vi "IMAQDevice.ReadIniFile.vi"(1 "ObjectName":string, 3 "Path":path, 5 "error in (no error)":errorcluster) -> (7 "Rotation":dbl, 8 "TimeOut":i32, 9 "Mirror":string, 10 "OffsetFromLeft":i32, 11 "HorizontalPixelPerMm":dbl, 12 "OffsetFromTop":i32, 13 "VerticalPixelPerMm":dbl, 14 "Serial Number":string, 15 "start sequence array":cluster{"Command":string, "Value":string}[](array[cluster]), 16 "Camera-Names":string[](array[string]), 17 "Grid":T1, 18 "GridR":T2, 19 "error out":errorcluster)   [LabVIEW 2014, in "IMAQDevice.lvlib"]
uses:
  IMAQDevice.lvlib
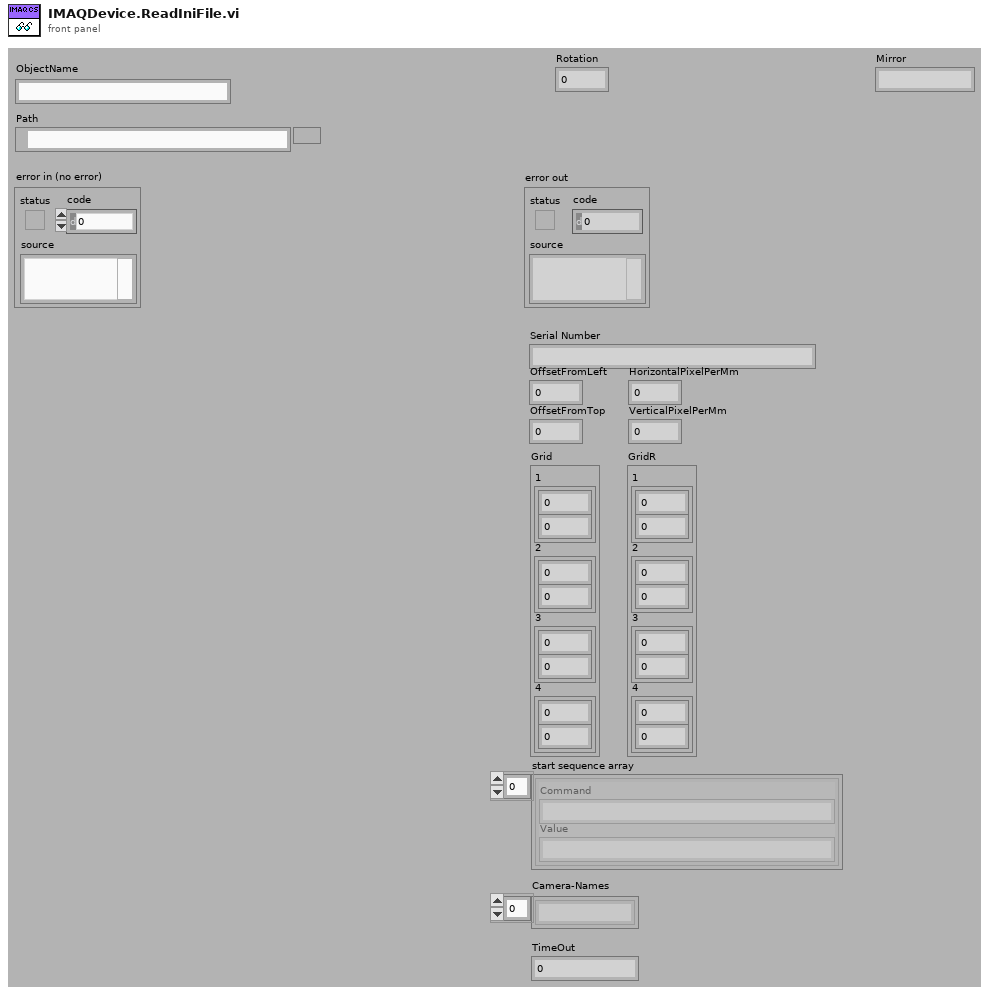
[diagram p1: front panel]
types:
  T1 = cluster{"1":cluster{i32, i32}, "2":cluster{i32, i32}, "3":cluster{i32, i32}, "4":cluster{i32, i32}}
  T2 = cluster{"1":cluster{dbl, dbl}, "2":cluster{dbl, dbl}, "3":cluster{dbl, dbl}, "4":cluster{dbl, dbl}}
  T3 = cluster{cluster{i32, i32}, cluster{i32, i32}, cluster{i32, i32}, cluster{i32, i32}}
  T4 = cluster{cluster{dbl, dbl}, cluster{dbl, dbl}, cluster{dbl, dbl}, cluster{dbl, dbl}}
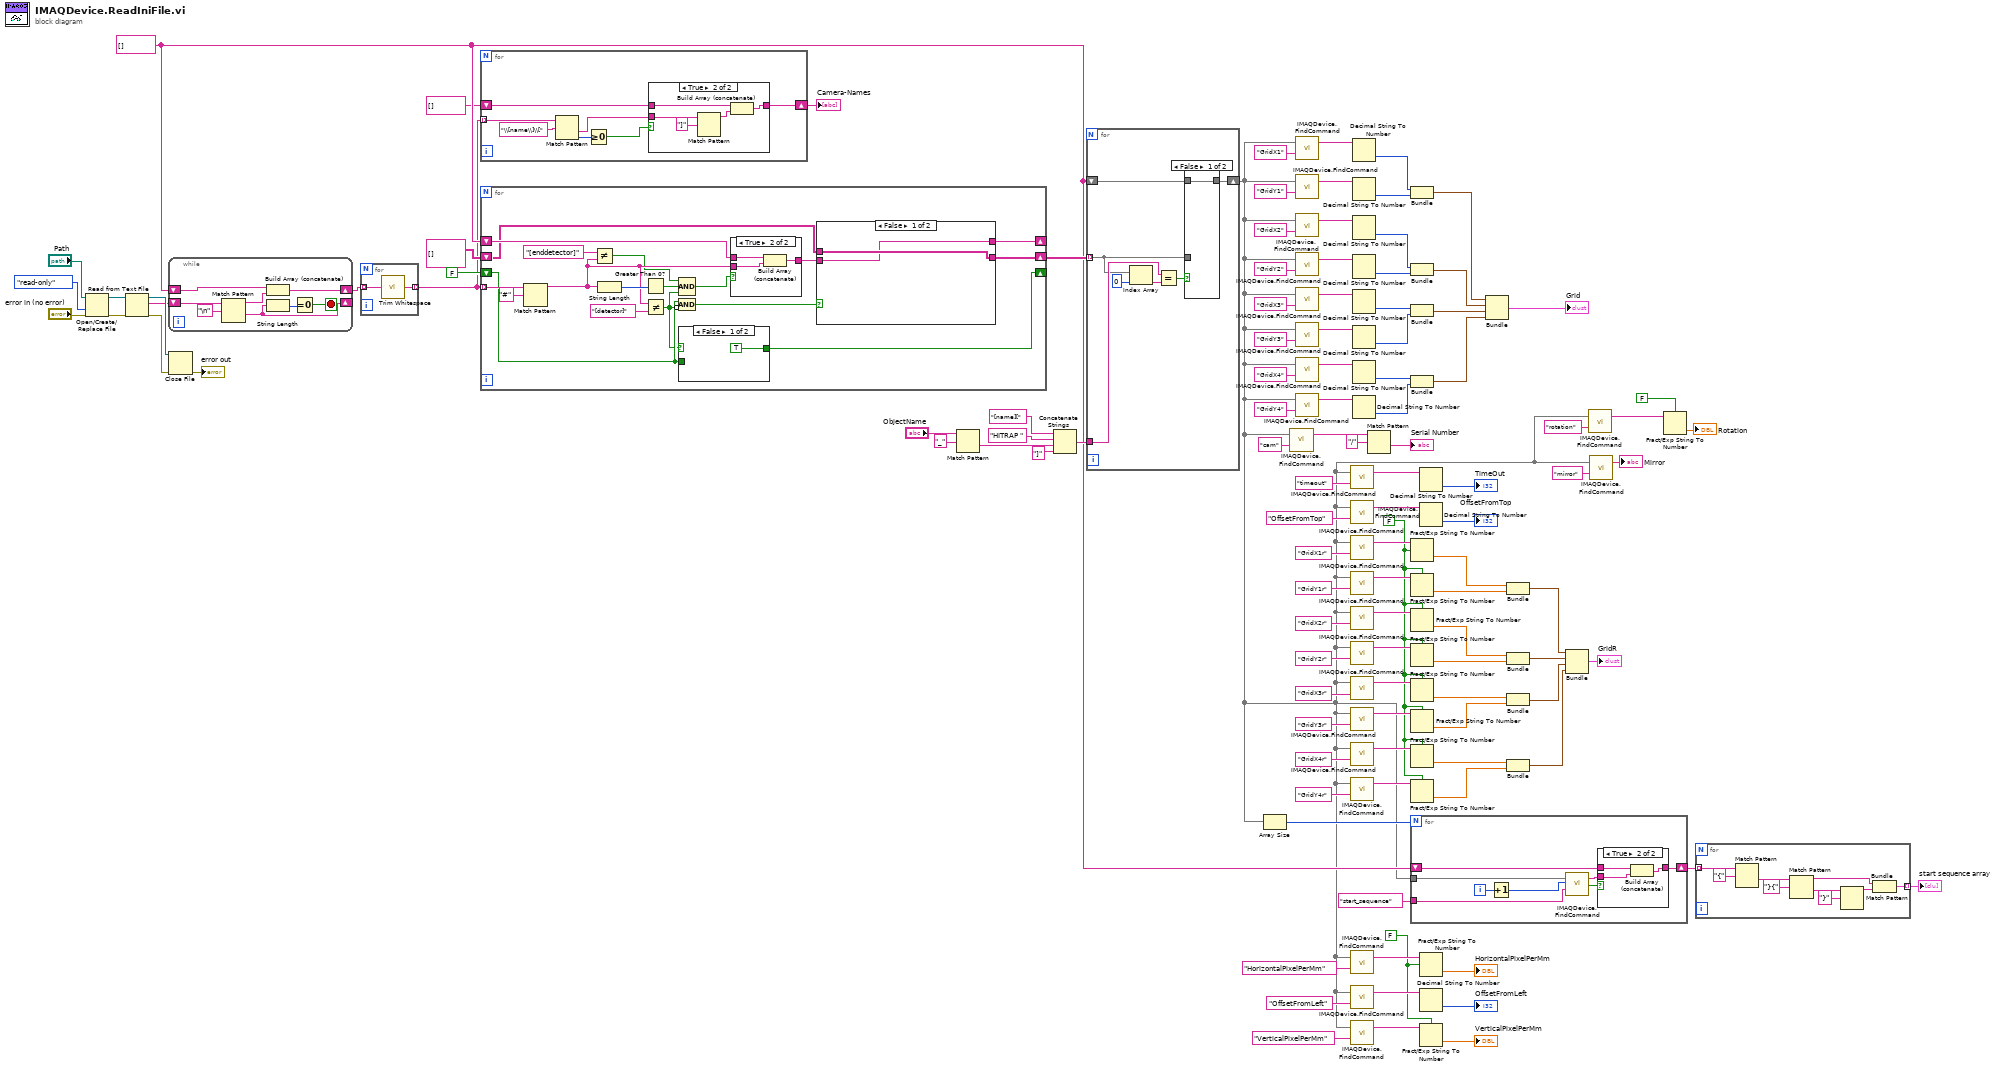
[diagram p0: block diagram]
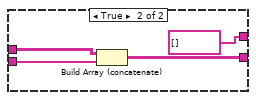
[diagram p6: hidden frame]
diagram:
  w8 = FALSE ("use system decimal point (T)")
  w9 = FALSE ("use system decimal point (T)")
  w27 = string[] []
  n1 = Open/Create/Replace File(file path (use dialog)="Path", error in="error in (no error)", access (0:read/write)=enum16{"read/write", "read-only", "write-only"}."read-only") -> (refnum out=w111:refnum<file>, error out=w110:errorcluster)  [unwired: 3 in, 1 out]
  n2 = Read from Text File(file (use dialog)=w111, error in=w110) -> (refnum out=w109:refnum<file>, text=w107:string, error out=w108:errorcluster)  [unwired: 2 in, 1 out]
  n3 = while {
    shift-right: [w117] -> _
    shift-left: w107 -> [w122]
    shift-right: [w119] -> w19
    shift-left: w27 -> [w120]
    stop <- w115 stop-if-true
    n4 = Match Pattern(string=w122, regular expression="\n") -> (before substring=w118:string, after substring=w117:string)  [unwired: 1 in, 2 out]
    n5 = Build Array (concatenate)(w120, w118) -> (w119:string[])
    n6 = String Length(string=w117) -> (length=w116:i32)
    n7 = Equal To 0?(x=w116) -> (x = 0?=w115:bool)
  }
  n8 = Close File(refnum=w109, error in=w108) -> (error out=→"error out":errorcluster)  [unwired: 1 out]
  n9 = for {
    tunnel: w19 -> [w124] mode=indexing
    tunnel: [w123] -> w18 mode=indexing
    n10 = call <vilib>:"Trim Whitespace.vi"("string"=w124) -> ("trimmed string"=w123:string)  [unwired: 1 in]
  }
  n11 = for {
    tunnel: w18 -> [w131] mode=indexing
    shift-right: [w128] -> w20
    shift-left: string[] [] -> [w129]
    n12 = Match Pattern(string=w131, regular expression="\\[name\\]\\[") -> (after substring=w126:string, offset past match=w127:i32)  [unwired: 1 in, 2 out]
    n13 = Greater Or Equal To 0?(x=w127) -> (x >= 0?=w125:bool)
    n14 = case shown="True" w125 {
      tunnel: w129 -> [w132 w137]
      tunnel: [w132 w136] -> w128
      tunnel: w126 -> [_ w134]
      frame False {
      }
      frame True {
        n15 = Match Pattern(string=w134, regular expression="]") -> (before substring=w133:string)  [unwired: 1 in, 3 out]
        n16 = Build Array (concatenate)(w137, w133) -> (w136:string[])
      }
    }
  }
  "Camera-Names" <- w20
  n17 = for {
    tunnel: w18 -> [w145] mode=indexing
    shift-right: [w147] -> w103
    shift-left: string[][] [] -> [w148]
    shift-right: [w144] -> _
    shift-left: w27 -> [w150]
    shift-right: [w143] -> _
    shift-left: FALSE -> [w142]
    n18 = Match Pattern(string=w145, regular expression="#") -> (before substring=w139:string)  [unwired: 1 in, 3 out]
    n19 = Not Equal?(x="[enddetector]" ("y"), y=w139) -> (x != y?=w138:bool)
    n20 = String Length(string=w139) -> (length=w155:i32)
    n21 = Greater Than 0?(x=w155) -> (x > 0?=w151:bool)
    n22 = Not Equal?(x=w139, y="[detector]") -> (x != y?=w141:bool)
    n23 = Compound Arithmetic op=AND(w138, w151, w141) -> (w152:bool)
    n24 = Compound Arithmetic op=AND(w142, invert w141) -> (w149:bool)
    n25 = case shown="False" w141 {
      tunnel: [TRUE w157] -> w143
      tunnel: w142 -> [_ w157]
      frame False {
      }
      frame True {
      }
    }
    n26 = case shown="True" w152 {
      tunnel: w139 -> [_ w167]
      tunnel: w150 -> [w164 w166]
      tunnel: [w164 w165] -> w146
      frame False {
      }
      frame True {
        n27 = Build Array (concatenate)(w166, w167) -> (w165:string[])
      }
    }
    n28 = case shown="False" w149 {
      tunnel: w148 -> [w159 w163]
      tunnel: [w159 w162] -> w147
      tunnel: w146 -> [w158 w161]
      tunnel: [w158 string[] []] -> w144
      frame False {
      }
      frame True {
        n29 = Build Array (concatenate)(w163, w161) -> (w162:string[][])
      }
    }
  }
  n30 = Match Pattern(string="ObjectName", regular expression="_") -> (after substring=w15:string)  [unwired: 1 in, 3 out]
  n31 = Concatenate Strings("[name][" ("string"), "HITRAP ", w15, "]" ("string")) -> (w102:string)
  n32 = for {
    tunnel: w103 -> [w169] mode=indexing
    tunnel: w102 -> [w172]
    shift-right: [w168] -> w4
    shift-left: w27 -> [w170]
    n33 = Index Array(array=w169, index=0) -> (element=w173:string)
    n34 = Equal?(x=w172, y=w173) -> (x = y?=w171:bool)
    n35 = case shown="False" w171 {
      tunnel: w170 -> [w175 _]
      tunnel: w169 -> [_ w176]
      tunnel: [w175 w176] -> w168
      frame False {
      }
      frame True {
      }
    }
  }
  n36 = Array Size(array=w4) -> (size(s)=w29:i32)
  n37 = call "IMAQDevice.FindCommand.vi"("Command Array"=w4, "Search String"="cam") -> ("Found Result"=w23:string)  [unwired: 16 in, 1 out]
  n38 = call "IMAQDevice.FindCommand.vi"("Command Array"=w4, "Search String"="GridX1") -> ("Found Result"=w79:string)  [unwired: 16 in, 1 out]
  n39 = call "IMAQDevice.FindCommand.vi"("Command Array"=w4, "Search String"="GridY1") -> ("Found Result"=w78:string)  [unwired: 16 in, 1 out]
  n40 = call "IMAQDevice.FindCommand.vi"("Command Array"=w4, "Search String"="GridX2") -> ("Found Result"=w77:string)  [unwired: 16 in, 1 out]
  n41 = call "IMAQDevice.FindCommand.vi"("Command Array"=w4, "Search String"="GridY2") -> ("Found Result"=w76:string)  [unwired: 16 in, 1 out]
  n42 = call "IMAQDevice.FindCommand.vi"("Command Array"=w4, "Search String"="GridX3") -> ("Found Result"=w75:string)  [unwired: 16 in, 1 out]
  n43 = call "IMAQDevice.FindCommand.vi"("Command Array"=w4, "Search String"="GridY3") -> ("Found Result"=w74:string)  [unwired: 16 in, 1 out]
  n44 = call "IMAQDevice.FindCommand.vi"("Command Array"=w4, "Search String"="GridX4") -> ("Found Result"=w73:string)  [unwired: 16 in, 1 out]
  n45 = call "IMAQDevice.FindCommand.vi"("Command Array"=w4, "Search String"="GridY4") -> ("Found Result"=w72:string)  [unwired: 16 in, 1 out]
  n46 = call "IMAQDevice.FindCommand.vi"("Command Array"=w4, "Search String"="timeout") -> ("Found Result"=w11:string)  [unwired: 16 in, 1 out]
  n47 = call "IMAQDevice.FindCommand.vi"("Command Array"=w4, "Search String"="OffsetFromTop") -> ("Found Result"=w96:string)  [unwired: 16 in, 1 out]
  n48 = call "IMAQDevice.FindCommand.vi"("Command Array"=w4, "Search String"="GridX1r") -> ("Found Result"=w50:string)  [unwired: 16 in, 1 out]
  n49 = call "IMAQDevice.FindCommand.vi"("Command Array"=w4, "Search String"="GridY1r") -> ("Found Result"=w49:string)  [unwired: 16 in, 1 out]
  n50 = call "IMAQDevice.FindCommand.vi"("Command Array"=w4, "Search String"="GridX2r") -> ("Found Result"=w48:string)  [unwired: 16 in, 1 out]
  n51 = call "IMAQDevice.FindCommand.vi"("Command Array"=w4, "Search String"="GridY2r") -> ("Found Result"=w47:string)  [unwired: 16 in, 1 out]
  n52 = call "IMAQDevice.FindCommand.vi"("Command Array"=w4, "Search String"="GridX3r") -> ("Found Result"=w46:string)  [unwired: 16 in, 1 out]
  n53 = call "IMAQDevice.FindCommand.vi"("Command Array"=w4, "Search String"="GridY3r") -> ("Found Result"=w45:string)  [unwired: 16 in, 1 out]
  n54 = call "IMAQDevice.FindCommand.vi"("Command Array"=w4, "Search String"="GridX4r") -> ("Found Result"=w44:string)  [unwired: 16 in, 1 out]
  n55 = call "IMAQDevice.FindCommand.vi"("Command Array"=w4, "Search String"="GridY4r") -> ("Found Result"=w43:string)  [unwired: 16 in, 1 out]
  n56 = call "IMAQDevice.FindCommand.vi"("Command Array"=w4, "Search String"="HorizontalPixelPerMm") -> ("Found Result"=w91:string)  [unwired: 16 in, 1 out]
  n57 = call "IMAQDevice.FindCommand.vi"("Command Array"=w4, "Search String"="OffsetFromLeft") -> ("Found Result"=w94:string)  [unwired: 16 in, 1 out]
  n58 = call "IMAQDevice.FindCommand.vi"("Command Array"=w4, "Search String"="VerticalPixelPerMm") -> ("Found Result"=w89:string)  [unwired: 16 in, 1 out]
  n59 = Decimal String To Number(string=w79) -> (number=w66:i32)  [unwired: 2 in, 1 out]
  n60 = Decimal String To Number(string=w78) -> (number=w65:i32)  [unwired: 2 in, 1 out]
  n61 = Decimal String To Number(string=w77) -> (number=w64:i32)  [unwired: 2 in, 1 out]
  n62 = Decimal String To Number(string=w76) -> (number=w63:i32)  [unwired: 2 in, 1 out]
  n63 = Decimal String To Number(string=w75) -> (number=w62:i32)  [unwired: 2 in, 1 out]
  n64 = Decimal String To Number(string=w74) -> (number=w61:i32)  [unwired: 2 in, 1 out]
  n65 = Decimal String To Number(string=w73) -> (number=w60:i32)  [unwired: 2 in, 1 out]
  n66 = Decimal String To Number(string=w72) -> (number=w59:i32)  [unwired: 2 in, 1 out]
  n67 = Match Pattern(string=w23, regular expression="/") -> (after substring=→"Serial Number":string)  [unwired: 1 in, 3 out]
  n68 = Bundle(w66, w65) -> (w70:cluster{i32, i32})  [unwired: 1 in]
  n69 = Bundle(w64, w63) -> (w69:cluster{i32, i32})  [unwired: 1 in]
  n70 = Bundle(w62, w61) -> (w68:cluster{i32, i32})  [unwired: 1 in]
  n71 = Bundle(w60, w59) -> (w67:cluster{i32, i32})  [unwired: 1 in]
  n72 = Fract/Exp String To Number(use system decimal point (T)=w9, string=w50) -> (number=w38:dbl)  [unwired: 2 in, 1 out]
  n73 = Fract/Exp String To Number(use system decimal point (T)=w9, string=w49) -> (number=w37:dbl)  [unwired: 2 in, 1 out]
  n74 = Fract/Exp String To Number(use system decimal point (T)=w9, string=w48) -> (number=w36:dbl)  [unwired: 2 in, 1 out]
  n75 = Fract/Exp String To Number(use system decimal point (T)=w9, string=w47) -> (number=w35:dbl)  [unwired: 2 in, 1 out]
  n76 = Fract/Exp String To Number(use system decimal point (T)=w9, string=w46) -> (number=w34:dbl)  [unwired: 2 in, 1 out]
  n77 = Fract/Exp String To Number(use system decimal point (T)=w9, string=w45) -> (number=w33:dbl)  [unwired: 2 in, 1 out]
  n78 = Fract/Exp String To Number(use system decimal point (T)=w9, string=w44) -> (number=w32:dbl)  [unwired: 2 in, 1 out]
  n79 = Fract/Exp String To Number(use system decimal point (T)=w9, string=w43) -> (number=w31:dbl)  [unwired: 2 in, 1 out]
  n80 = for {
    N: w29 -> [_]
    tunnel: w4 -> [w184]
    tunnel: "start_sequence" ("Search String") -> [w181]
    shift-right: [w178] -> w26
    shift-left: w27 -> [w179]
    i -> [w183]
    n81 = Increment(x=w183) -> (x+1=w182:i32)
    n82 = call "IMAQDevice.FindCommand.vi"("Command Array"=w184, "Sequence Number"=w182, "Search String"=w181) -> ("Found Result"=w177:string, "Found?"=w180:bool)  [unwired: 15 in]
    n83 = case shown="True" w180 {
      tunnel: w179 -> [w185 w187]
      tunnel: [w185 w188] -> w178
      tunnel: w177 -> [_ w186]
      frame False {
      }
      frame True {
        n84 = Build Array (concatenate)(w187, w186) -> (w188:string[])
      }
    }
  }
  n85 = Decimal String To Number(string=w11) -> (number=→"TimeOut":i32)  [unwired: 2 in, 1 out]
  n86 = Decimal String To Number(string=w96) -> (number=→"OffsetFromTop":i32)  [unwired: 2 in, 1 out]
  n87 = Fract/Exp String To Number(use system decimal point (T)=w8, string=w91) -> (number=→"HorizontalPixelPerMm":dbl)  [unwired: 2 in, 1 out]
  n88 = Decimal String To Number(string=w94) -> (number=→"OffsetFromLeft":i32)  [unwired: 2 in, 1 out]
  n89 = Fract/Exp String To Number(use system decimal point (T)=w8, string=w89) -> (number=→"VerticalPixelPerMm":dbl)  [unwired: 2 in, 1 out]
  n90 = Bundle(w70, w69, w68, w67) -> (→"Grid":T3)  [unwired: 1 in]
  n91 = Bundle(w38, w37) -> (w42:cluster{dbl, dbl})  [unwired: 1 in]
  n92 = Bundle(w36, w35) -> (w41:cluster{dbl, dbl})  [unwired: 1 in]
  n93 = Bundle(w34, w33) -> (w40:cluster{dbl, dbl})  [unwired: 1 in]
  n94 = Bundle(w32, w31) -> (w39:cluster{dbl, dbl})  [unwired: 1 in]
  n95 = Bundle(w42, w41, w40, w39) -> (→"GridR":T4)  [unwired: 1 in]
  n96 = call "IMAQDevice.FindCommand.vi"("Command Array"=w4, "Search String"="rotation") -> ("Found Result"=w3:string)  [unwired: 16 in, 1 out]
  n97 = call "IMAQDevice.FindCommand.vi"("Command Array"=w4, "Search String"="mirror") -> ("Found Result"=→"Mirror":string)  [unwired: 16 in, 1 out]
  n98 = Fract/Exp String To Number(use system decimal point (T)=FALSE, string=w3) -> (number=→"Rotation":dbl)  [unwired: 2 in, 1 out]
  n99 = for {
    tunnel: w26 -> [w197] mode=indexing
    tunnel: [w189] -> w25 mode=indexing
    n100 = Match Pattern(string=w197, regular expression="{") -> (after substring=w195:string)  [unwired: 1 in, 3 out]
    n101 = Match Pattern(string=w195, regular expression="}{") -> (before substring=w191:string, after substring=w193:string)  [unwired: 1 in, 2 out]
    n102 = Match Pattern(string=w193, regular expression="}") -> (before substring=w190:string)  [unwired: 1 in, 3 out]
    n103 = Bundle(w191, w190) -> (w189:cluster{string, string})  [unwired: 1 in]
  }
  "start sequence array" <- w25
